vi "RIGOL DS1000 Series Acquire Multiple Waveforms.vi"() -> ()   [LabVIEW 2017]
doc: "This example shows how to configure multiple channels and acquire waveforms from multiple channels."
uses:
  <instrlib>/RIGOL DS1000 Series/Public/Data/Read (Multiple Waveforms).vi
panel:
  in  "Channel B(1: Channel 1)":u16(ring)=1 items=["Channel 1"=1, "Channel 2"=2]
  in  "Channel A(1: Channel 1)":u16(ring)=1 items=["Channel 1"=1, "Channel 2"=2]
  in  "Vertical Coupling B (1: DC)":u16(ring)=1 items=["AC", "DC", "Ground"]
  in  "Vertical Coupling A(1: DC)":u16(ring)=1 items=["AC", "DC", "Ground"]
  in  "Timeout (10000 ms)":u32=10000
  out "Waveform Data":waveform(dbl)[](graph)
  in  "VISA resource name":refnum<visa-resource-name>
  # "(c) 2010-2012, RIGOL Technologies, Inc.  All Rights Reserved."
  # "Channel A"
  # "Channel B"
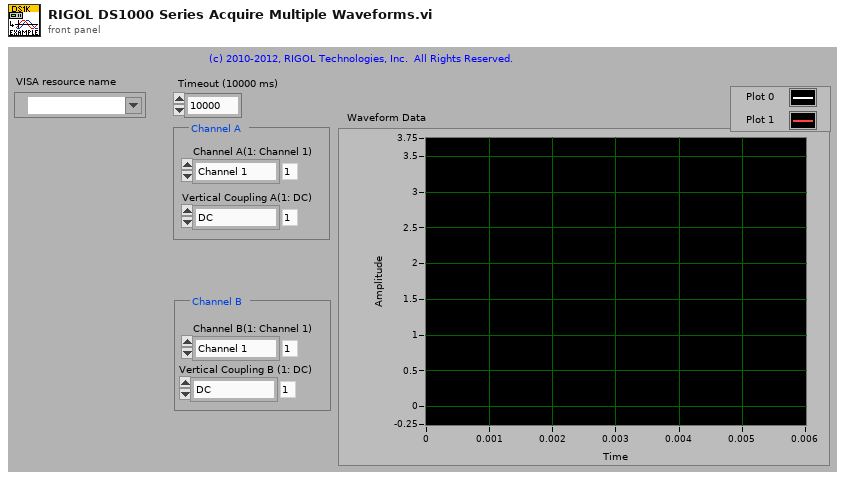
[diagram p1: front panel]
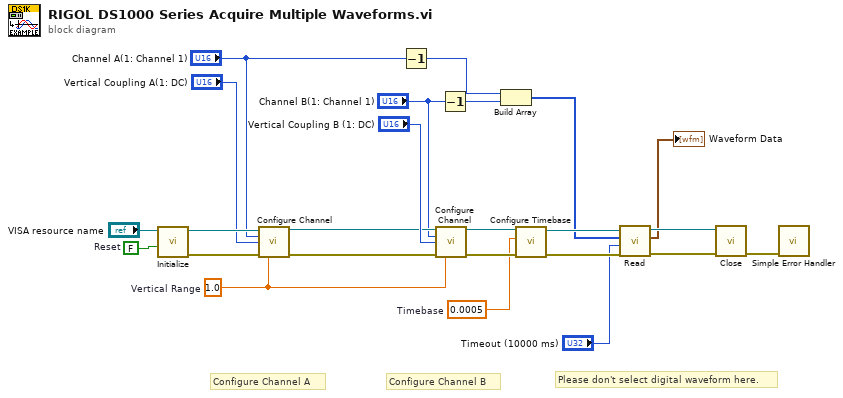
[diagram p0: block diagram]
diagram:
  w5 = FALSE  # Reset
  w12 = 1.0  # Vertical Range
  w11 = 0.0005  # Timebase
  # "Please don't select digital waveform here."
  # "Configure Channel B"
  # "Configure Channel A"
  n1 = call <instrlib>:"Initialize.vi"("Reset (True)"=w5, "VISA resource name"="VISA resource name") -> ("error out"=w19:errorcluster, "VISA resource name out"=w20:refnum<visa-resource-name>)  [unwired: 2 in, 6 out]
  n2 = call <instrlib>:"Configure Channel.vi"("VISA resource name"=w20, "Channel (1: Channel 1)"="Channel A(1: Channel 1)", "Vertical Coupling (0: DC)"="Vertical Coupling A(1: DC)", "error in (no error)"=w19, "Vertical Range (1.0 V)"=w12) -> ("VISA resource name out"=w8:refnum<visa-resource-name>, "error out"=w7:errorcluster)  [unwired: 3 in, 6 out]
  n3 = Decrement(x="Channel A(1: Channel 1)") -> (x-1=w1:u16)
  n4 = call <instrlib>:"Configure Channel.vi"("VISA resource name"=w8, "Channel (1: Channel 1)"="Channel B(1: Channel 1)", "Vertical Coupling (0: DC)"="Vertical Coupling B (1: DC)", "error in (no error)"=w7, "Vertical Range (1.0 V)"=w12) -> ("VISA resource name out"=w18:refnum<visa-resource-name>, "error out"=w17:errorcluster)  [unwired: 3 in, 6 out]
  n5 = Decrement(x="Channel B(1: Channel 1)") -> (x-1=w2:u16)
  n6 = Build Array(w1, w2) -> (w6:u16[])
  n7 = call <instrlib>:"Configure Timebase.vi"("error in (no error)"=w17, "Timebase (0.0005 s)"=w11, "VISA resource name"=w18) -> ("error out"=w15:errorcluster, "VISA resource name out"=w16:refnum<visa-resource-name>)  [unwired: 1 in, 6 out]
  n8 = call-poly <instrlib>:"Read.vi"("error in (no error)"=w15, "Timeout (10000 ms)"="Timeout (10000 ms)", "Channels"=w6, "VISA resource name"=w16) -> ("error out"=w21:errorcluster, "Waveform Data"=→"Waveform Data":waveform(dbl)[], "VISA resource name out"=w22:refnum<visa-resource-name>)  [unwired: 5 out]
  n9 = call <instrlib>:"Close.vi"("error in (no error)"=w21, "VISA resource name"=w22) -> ("error out"=w23:errorcluster)  [unwired: 9 out]
  n10 = call <vilib>:"Simple Error Handler.vi"("error in (no error)"=w23) -> ()  [unwired: 1 in, 8 out]
